vi "pcfs_format_chart.vi"(8 "error in (no error)":errorcluster, 10 "info":T1, 11 "scan_panel in":refnum<class "pcfs.lvclass">) -> (0 "error out":errorcluster, 3 "panel out":refnum<class "pcfs.lvclass">)   [LabVIEW 2015, in "pcfs.lvclass"]
uses:
  pcfs.lvclass
  Scan/scan_hdf5_log/initialization_data.ctl
  <vilib>/Utility/miscctls.llb/LVOffsetAndMultiplierTypeDef.ctl
  UI/panel_class/panel.lvclass/panel.ctl
  UI/panel_class/panel.lvclass
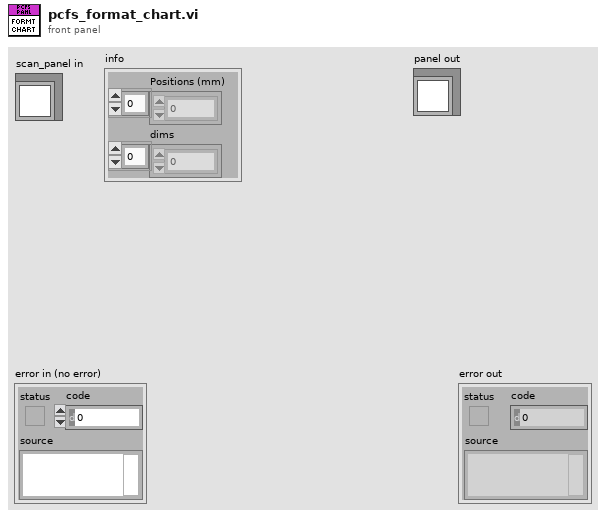
[diagram p1: front panel]
types:
  T1 = typedef "initialization_data.ctl" = cluster{"Positions (mm)":dbl[], "dims":u32[]}
  T2 = typedef "LVOffsetAndMultiplierTypeDef.ctl" = cluster{"Offset":dbl, "Multiplier":dbl}
  T3 = typedef "ui_plot_references.ctl" = cluster{"plots":refnum<vi>, "chart":refnum<vi>, "graph":refnum<vi>, "map":refnum<vi>, "XY Graph":refnum<vi>}
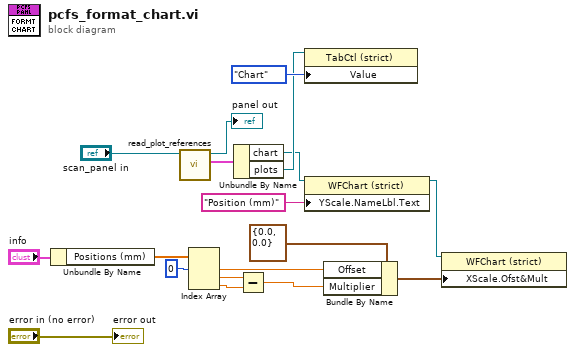
[diagram p0: block diagram]
diagram:
  n1 = Unbundle By Name("info") -> ("Positions (mm)"=w2:dbl[])
  n2 = call "read_plot_references.vi"("panel in"="scan_panel in") -> ("plot_references"=w14:T3, "panel out"=→"panel out":refnum<class "pcfs.lvclass">)  [unwired: 8 in, 1 out]
  n3 = Index Array(array=w2, index #1=0 ("index")) -> (element #1=w7:dbl, element #2=w8:dbl, element #3=w6:dbl)  [unwired: 2 in]
  n4 = Unbundle By Name(w14) -> ("chart"=w1:refnum<vi>, "plots"=w16:refnum<vi>)
  n5 = Subtract(x=w8, y=w6) -> (x-y=w5:dbl)
  n6 = property class="TabCtl (strict)"(reference=w16, "Value"=enum32{"Chart", "Graph", "Map", "XY Graph"}."Chart") -> ()  [unwired: 1 in, 2 out]
  n7 = property class="WFChart (strict)"(reference=w1, "YScale.NameLbl.Text"="Position (mm)" ("Y Scale.Name Label.Text")) -> (reference out=w12:refnum<vi>)  [unwired: 1 in, 1 out]
  n8 = Bundle By Name(cluster=T2 {"Offset"=0.0, "Multiplier"=0.0} ("X Scale.Offset and Multiplier"), "Offset"=w7, "Multiplier"=w5) -> (w10:T2)
  n9 = property class="WFChart (strict)"(reference=w12, "XScale.Ofst&Mult"=w10) -> ()  [unwired: 1 in, 2 out]
  "error out" <- "error in (no error)"
